vi "process_document.vi"(0 "embed_nodes in":refnum<class "embed_nodes.lvclass">, 5 "documents":refnum<class "data_document.lvclass">[](array[class]), 11 "error in (no error)":errorcluster) -> (4 "embed_nodes out":refnum<class "embed_nodes.lvclass">, 6 "nodes":refnum<class "data_node.lvclass">[](array[class]), 15 "error out":errorcluster)   [LabVIEW 2020, in "embed_nodes.lvclass"]
uses:
  embed_nodes.lvclass
  data/data_document/data_document.lvclass
  data/data_node/data_node.lvclass
  embed_nodes.lvclass/embed_nodes.ctl
  models/message_text/message_text.lvclass
  D:/Personal/LabVIEW LLMs/src/models/abstract_message_base/abstract_message_base.lvclass
  models/message_vectors/message_vectors.lvclass
  models/abstract_llm_embedding/abstract_llm_embedding.lvclass
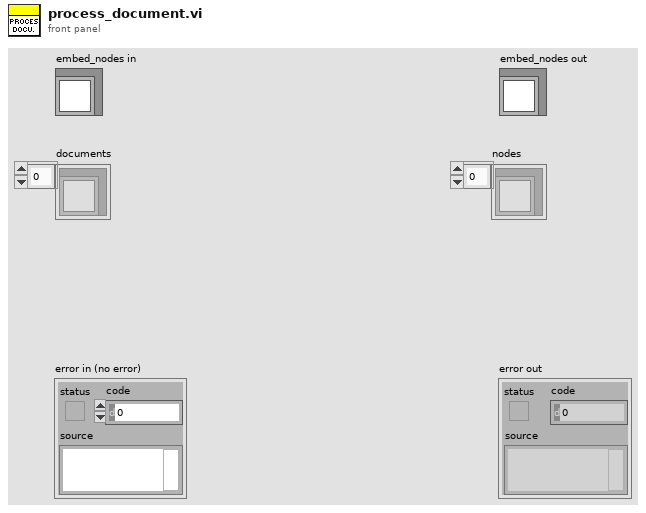
[diagram p1: front panel]
types:
  T1 = typedef "message_vectors.lvclass/embedding.ctl" = cluster{"index":u32, "Vectors":dbl[]}
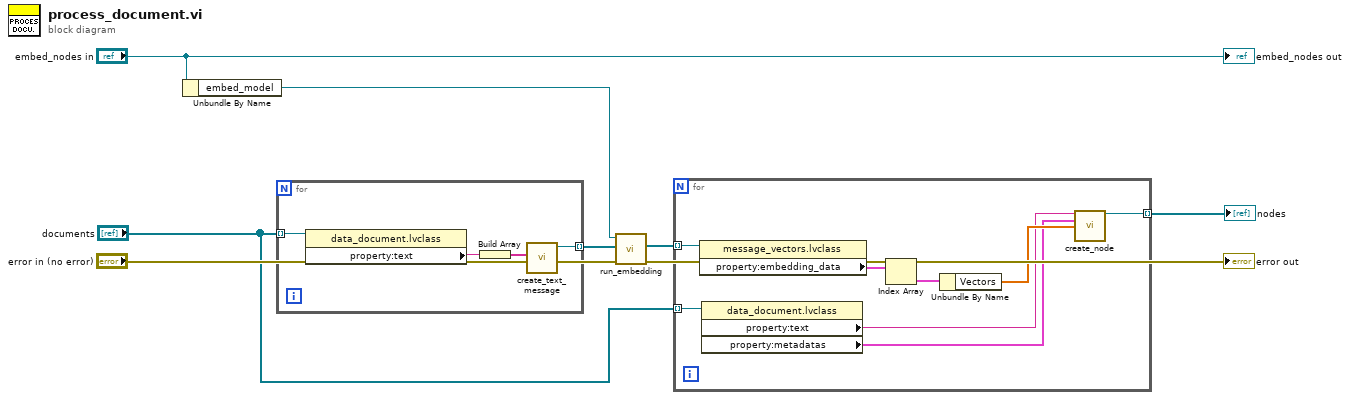
[diagram p0: block diagram]
diagram:
  n1 = Unbundle By Name("embed_nodes in") -> ("embed_model"=w7:refnum<class "abstract_llm_base.lvclass">)
  n2 = for {
    tunnel: "documents" -> [w12] mode=indexing
    tunnel: [w9] -> w6 mode=indexing
    n3 = property class="data_document.lvclass"(reference=w12) -> ("property:text"=w11:string)  [unwired: 1 in, 2 out]
    n4 = Build Array(w11) -> (w10:string[])
    n5 = call "create_text_message.vi"("content"=w10) -> ("message_text out"=w9:refnum<class "message_text.lvclass">)  [unwired: 9 in, 1 out]
  }
  n6 = call "run_embedding.vi"("error in (no error)"="error in (no error)", "Messages"=w6, "abstract_llm_embedding in"=w7) -> ("error out"=→"error out":errorcluster, "Response"=w4:refnum<class "message_vectors.lvclass">[])  [unwired: 6 in, 1 out]
  n7 = for {
    tunnel: w4 -> [w20] mode=indexing
    tunnel: "documents" -> [w16] mode=indexing
    tunnel: [w13] -> w2 mode=indexing
    n8 = property class="message_vectors.lvclass"(reference=w20) -> ("property:embedding_data"=w19:T1[])  [unwired: 1 in, 2 out]
    n9 = property class="data_document.lvclass"(reference=w16) -> ("property:text"=w15:string, "property:metadatas"=w14:cluster{"key":string, "value":string}[])  [unwired: 1 in, 2 out]
    n10 = Index Array(array=w19) -> (element=w18:T1)  [unwired: 1 in]
    n11 = Unbundle By Name(w18) -> ("Vectors"=w17:dbl[])
    n12 = call "create_node.vi"("text"=w15, "metadatas"=w14, "vector"=w17) -> ("data_node out"=w13:refnum<class "data_node.lvclass">)  [unwired: 11 in, 1 out]
  }
  "nodes" <- w2
  "embed_nodes out" <- "embed_nodes in"
